vi "Voltage DAQ 07-06-2023 Current version.vi"() -> ()   [LabVIEW 2022 SP3]
uses:
  <vilib>/Utility/file.llb/Read Delimited Spreadsheet (string).vi
  <vilib>/Utility/file.llb/Write Delimited Spreadsheet (string).vi
  Labview 2018/Sub Vi's/Tektronix DPO MSO 2000 4000 Series.lvlib
panel:
  in  "Amplitude measurements":enum16{"Only test segment", "Every segment"}(ring)
  in  "Min Power (uW)":dbl=1.4
  in  "Ramping or Constant Current":enum16{"Ramping Current", "Constant Current"}(ring)
  in  "Numbers of tests":dbl
  out "Segments Run":string
  out "Power List (W)":string[](array[string])
  in  "Max Power (uW)":dbl=1200.0
  in  "Max index Seg 1 (= #Steps-1)":dbl=59.0
  out "Bandwidth":dbl[](graph)
  out "Read Buffer 2":string
  out "Read Buffer":string="+8.16433198379414E-11 ,+1.36474786384321E-14 ,+7.54655698703987E-02 ,+2.55183753967285E+01 ,+4.95928985373852E+06 ,+0.00000000000000E+00 ,+4.95929057417896E+06 ,+4.95926294501331E+06 ,+4.95931676260974E+06 \n"
  out "Local":dbl(slide) scale=0.0..100.0
  in  "Test Control":T1(ring)
  out "Ch2 Meas 2":dbl
  out "Ch1 Meas 2":dbl
  in  "Voltage Stabilize Wait (s)":dbl=1.0
  out "Ch 2 (Measurement 2)":dbl[](graph)
  out "Ch 1 (Measurement 2)":dbl[](graph)
  out "Ch2 Meas 1":dbl
  in  "Measurement 2":i32(ring)=21 items=["Period", "Frequency", "Delay", "Rise Time", "Fall Time", "Positive Duty Cycle", "Negative Duty Cycle", "Positive Pulse Width", "Negative Pulse Width", "Burst Width", "Phase", "Positive Overshoot", "Negative Overshoot", "Vpp", "Amplitude", "Voltage High", "Voltage Low", "Voltage Max", "Voltage Min", "Voltage Mean", "Voltage Mean (cycle)", "Voltage RMS", "Voltage RMS (cycle)", "Area", "Cycle Area", "Positive Edge Count", "Negative Edge Count", "Positive Pulse Count", "Negative Pulse Count", "Total Overshoot"]
  out "Ch1 Meas 1":dbl
  in  "Measurement 1":i32(ring)=13 items=["Period", "Frequency", "Delay", "Rise Time", "Fall Time", "Positive Duty Cycle", "Negative Duty Cycle", "Positive Pulse Width", "Negative Pulse Width", "Burst Width", "Phase", "Positive Overshoot", "Negative Overshoot", "Vpp", "Amplitude", "Voltage High", "Voltage Low", "Voltage Max", "Voltage Min", "Voltage Mean", "Voltage Mean (cycle)", "Voltage RMS", "Voltage RMS (cycle)", "Area", "Cycle Area", "Positive Edge Count", "Negative Edge Count", "Positive Pulse Count", "Negative Pulse Count", "Total Overshoot"]
  out "Global":u8(slide) scale=0.0..100.0
  out "Power (uW)":dbl
  out "Index (=Step#-1)":dbl=108.0
  out "Frequency":dbl[](graph)=[4959289.62588808, 4959289.85373852]
  in  "Sweep Time (s)":dbl=1.0
  in  "Step Next":bool
  in  "stop":bool
  in  "Pause":bool
  in  "Test Instructions":string="Note - DPO RESOURCE IS 11856 not 11850\nOscilloscope: Set Ch1 to 50mV (powers<80uW) or 100mV (powers between 80 and 400uW) or 200mV (powers>400uW). \nSet Ch 2 to 20 mV. \nSet trigger to 0V on  CH 1.\n"
  in  "Notes":string="Tip is 100um Stainless Steel"
  in  "Sample":string="DLC"
  in  "Sample Number":string="Box 5b Xtal 1"
  in  "Load":string="50 uN"
  in  "Tip Number":string="H10 "
  in  "Test Name":string="Ramp 3 Loc 9 test 001"
  in  "Humidity":string="2.2%"
  in  "Date":string="10/10/2022"
  in  "DPO2014 VISA Resource Name":refnum<visa-resource-name>="USB0::0x0699::0x0373::C011856::INSTR"
  in  "E5100A VISA Resource Name":refnum<visa-resource-name>="GPIB0::17::INSTR"
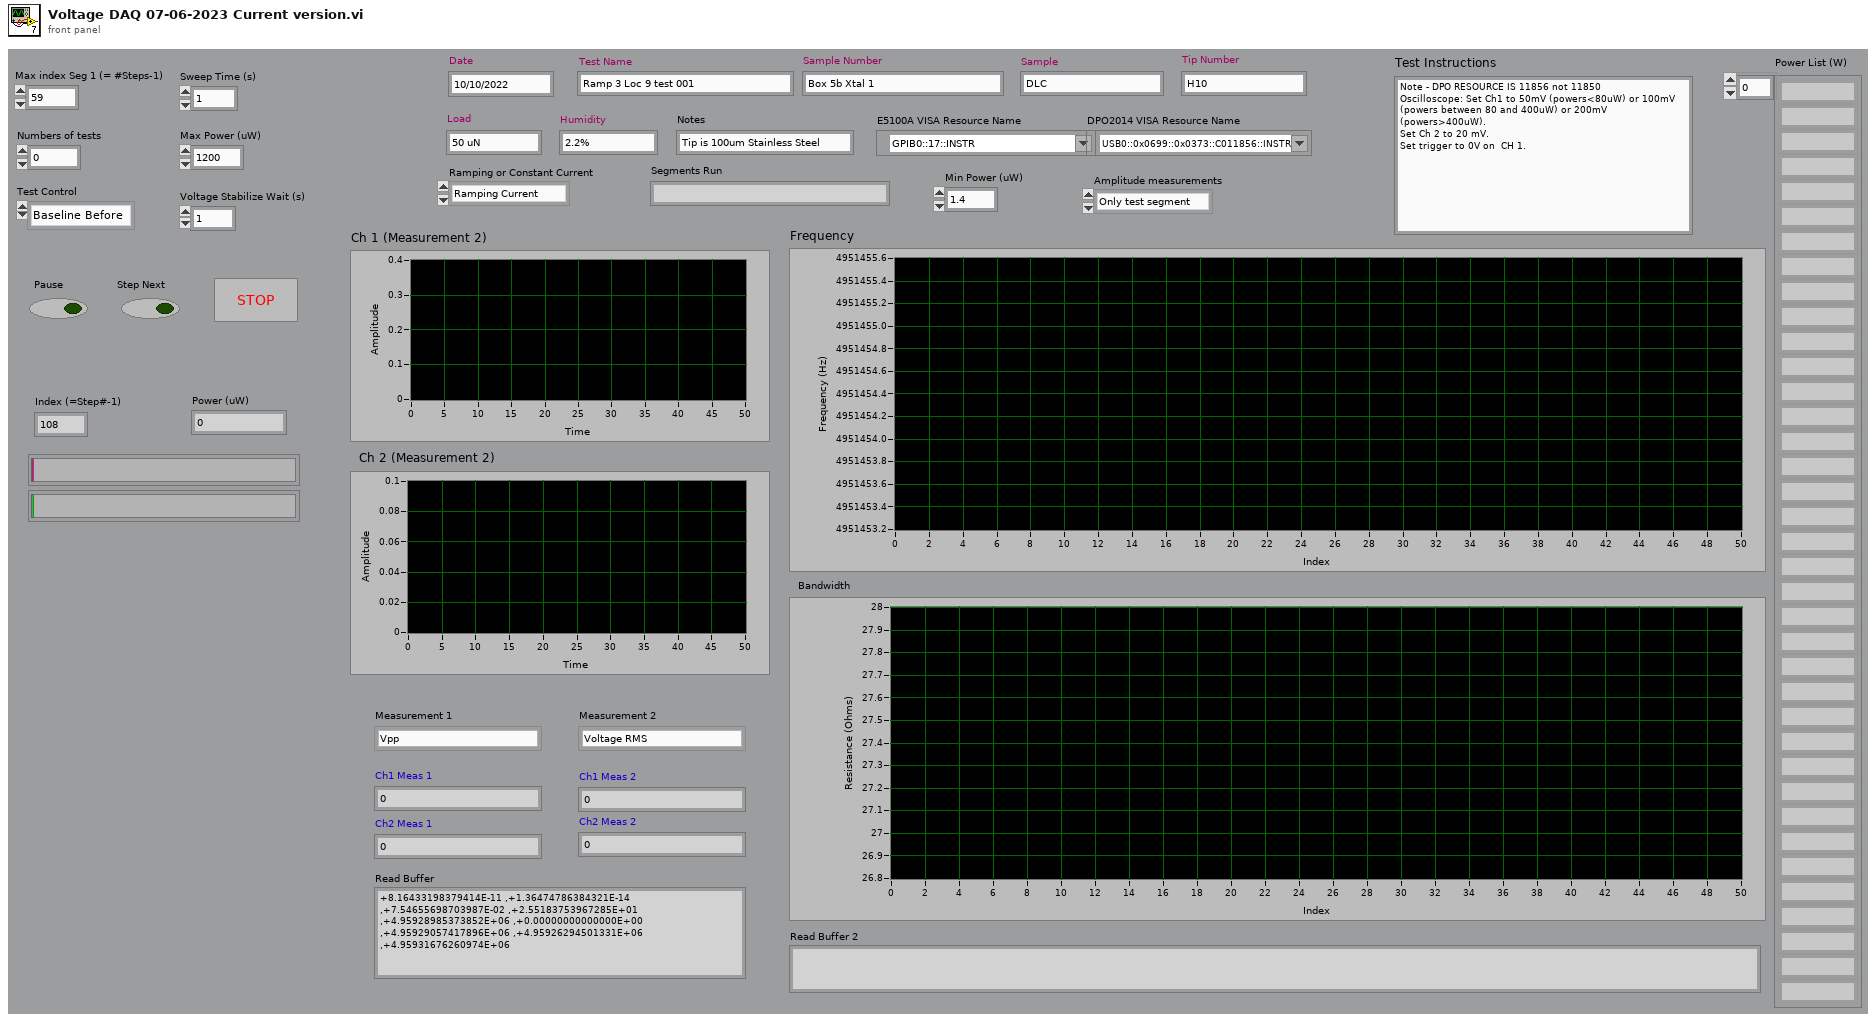
[diagram p1: front panel]
types:
  T1 = enum16{"Baseline Before", "Run-in", "Test", "Baseline After"}
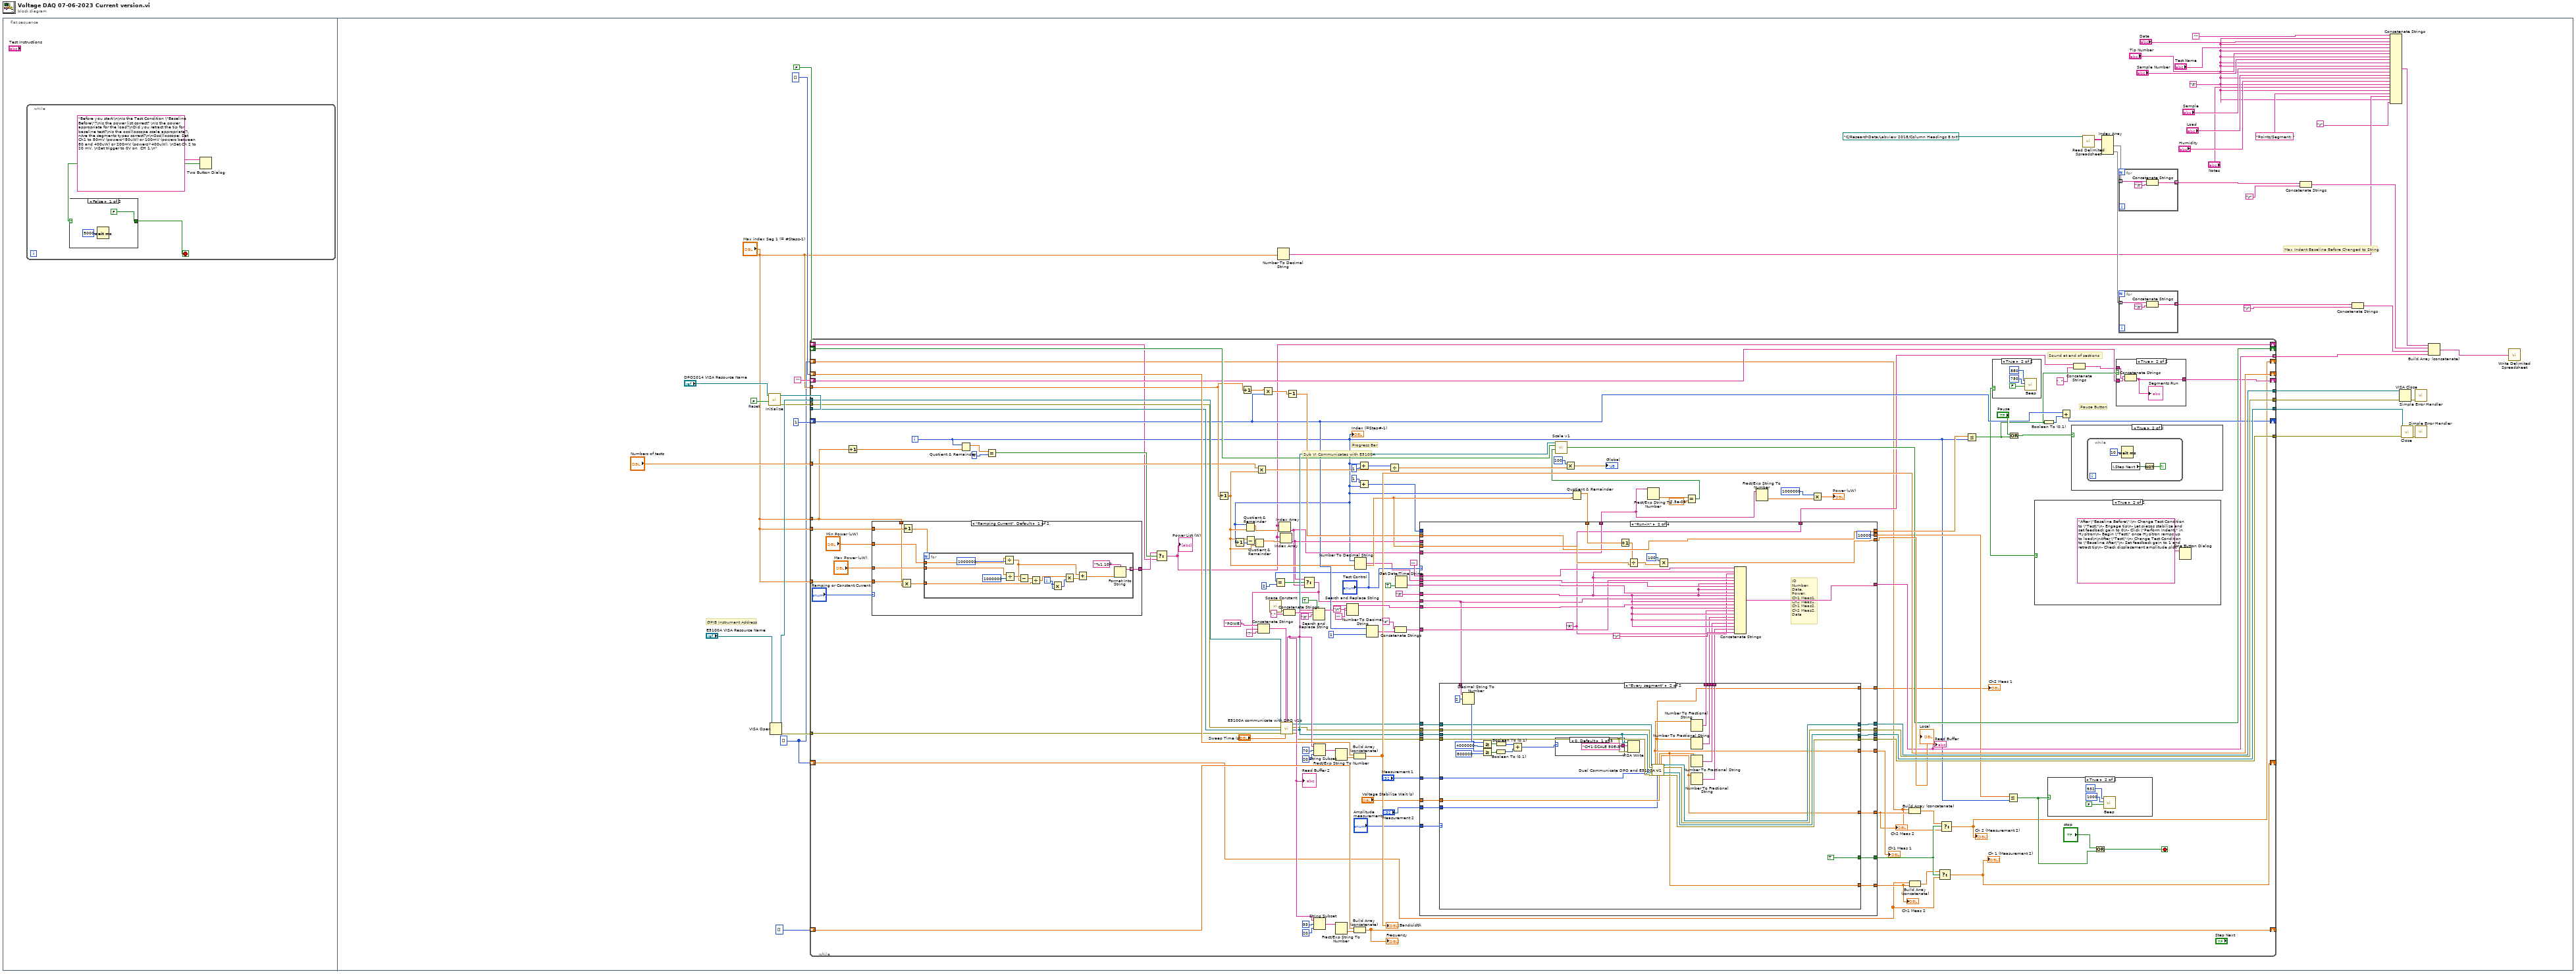
[diagram p0: block diagram]
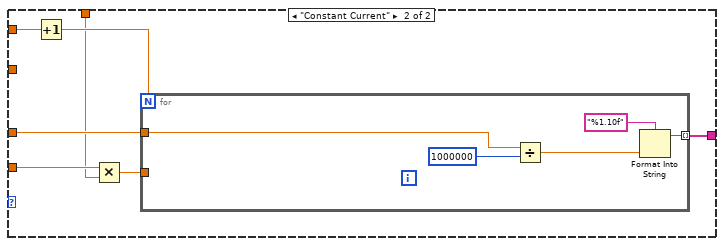
[diagram p3: hidden frame]
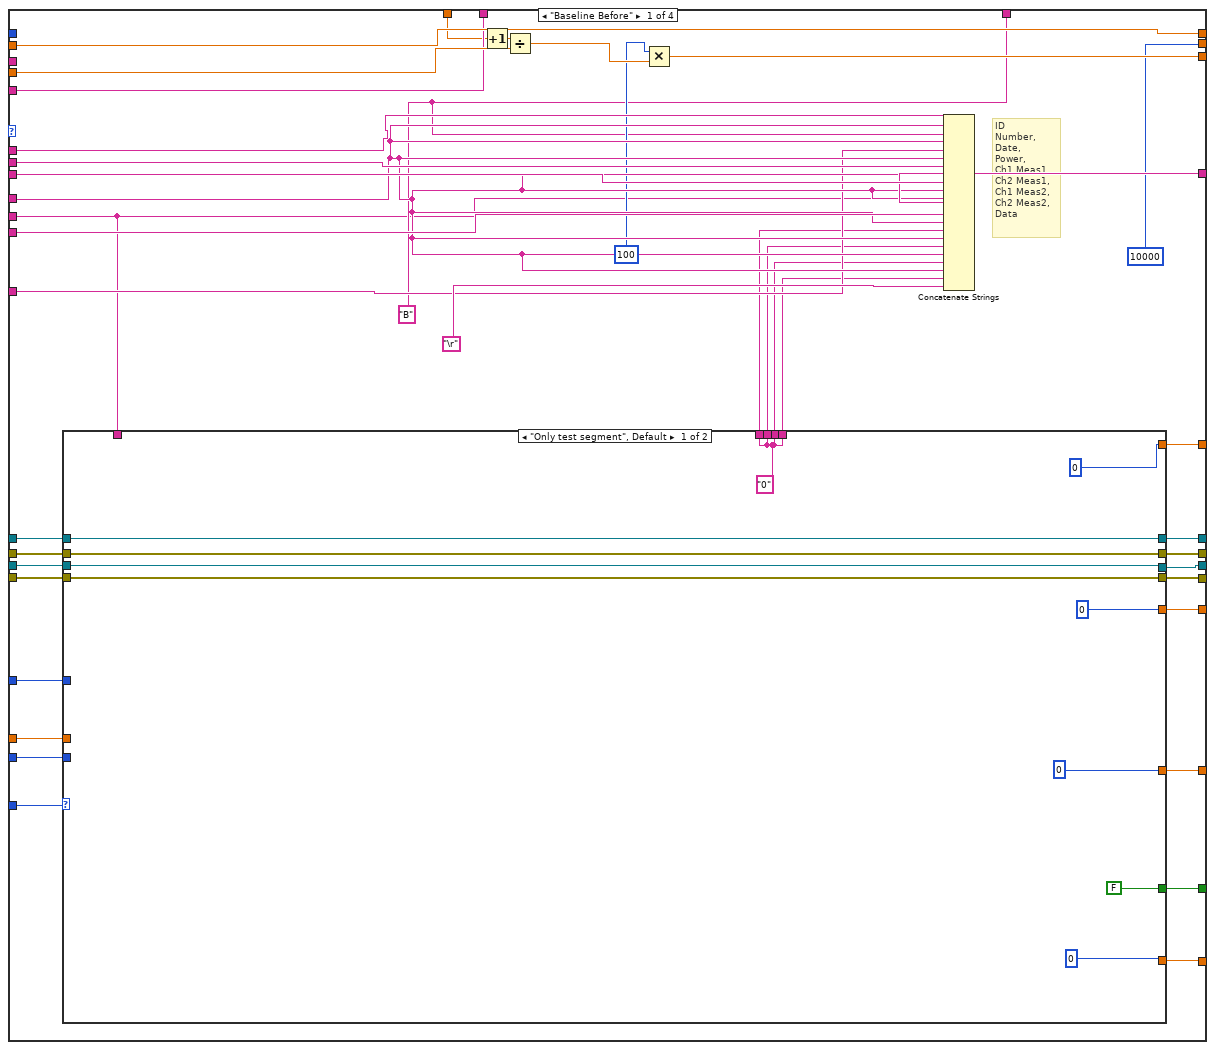
[diagram p8: hidden frame]
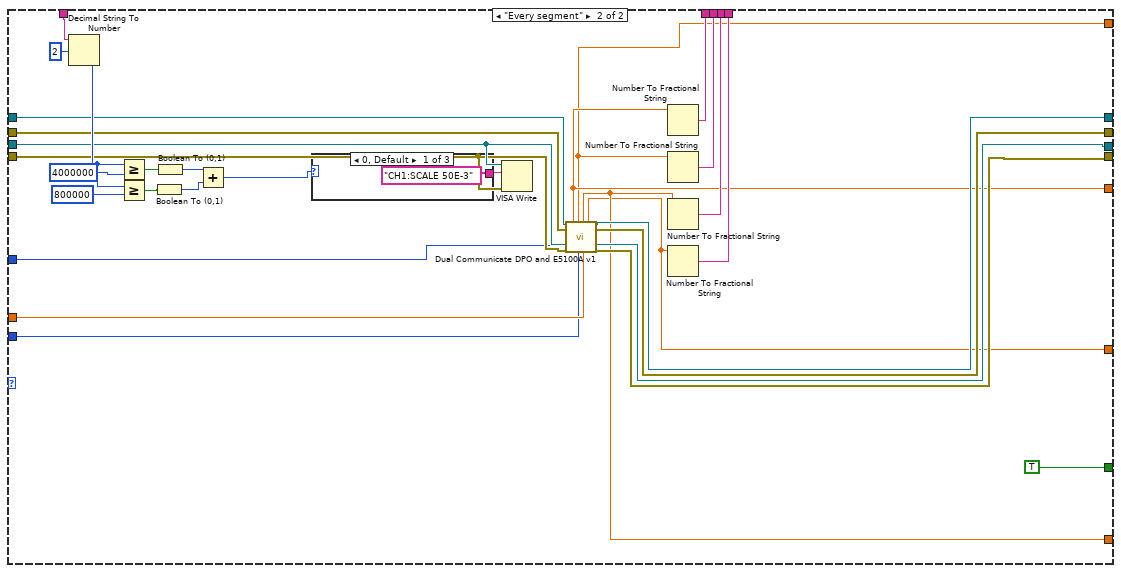
[diagram p9: hidden frame]
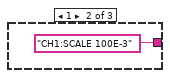
[diagram p10: hidden frame]
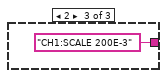
[diagram p11: hidden frame]
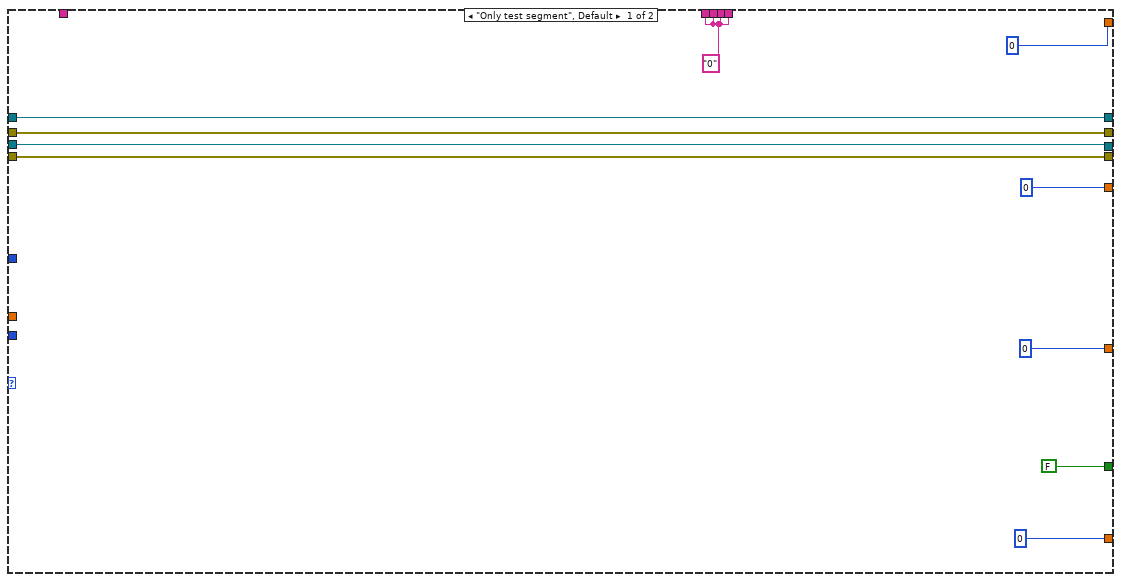
[diagram p12: hidden frame]
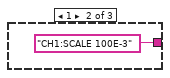
[diagram p13: hidden frame]
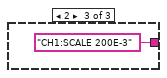
[diagram p14: hidden frame]
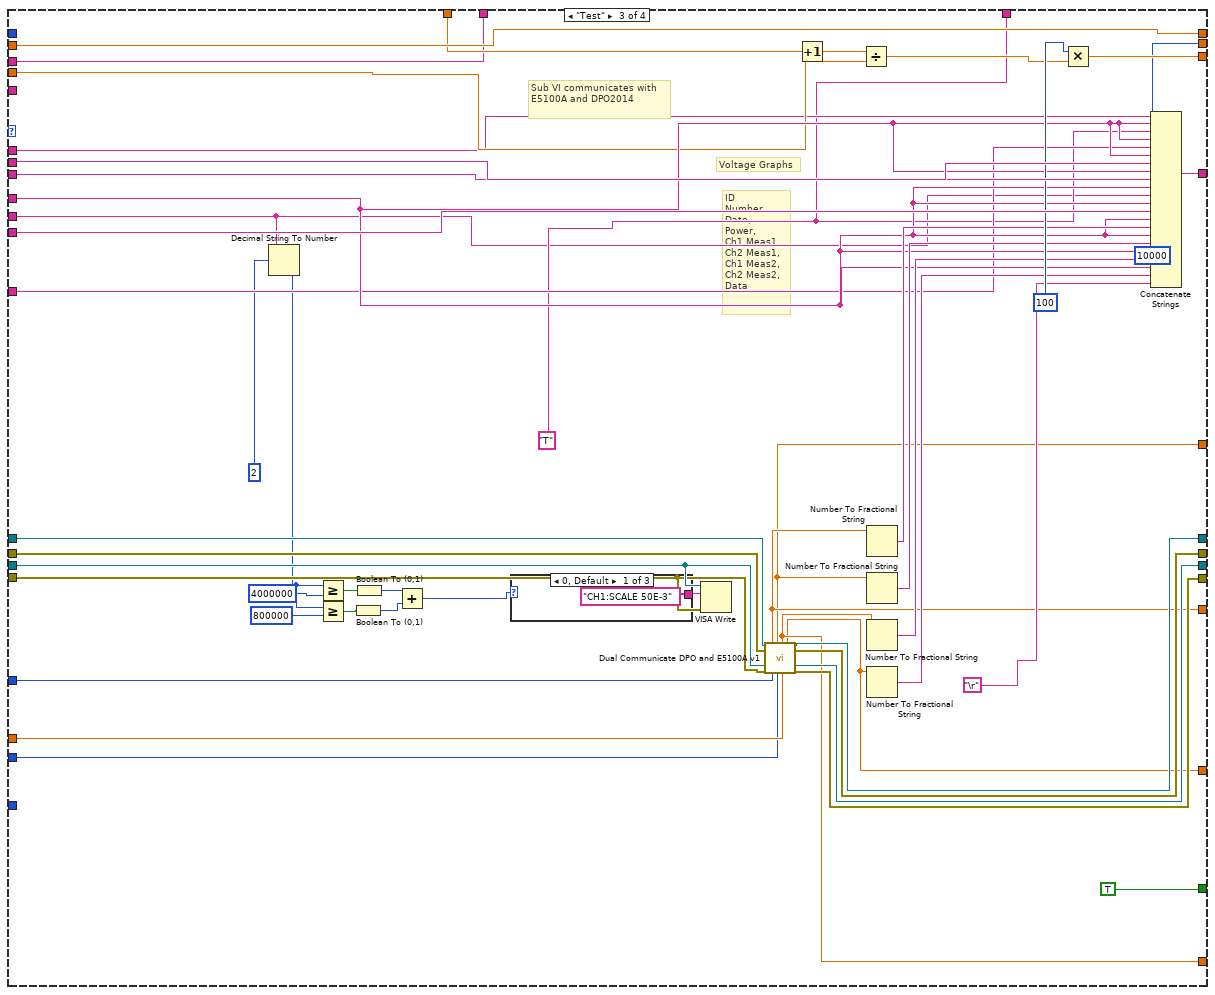
[diagram p15: hidden frame]
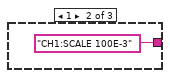
[diagram p16: hidden frame]
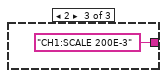
[diagram p17: hidden frame]
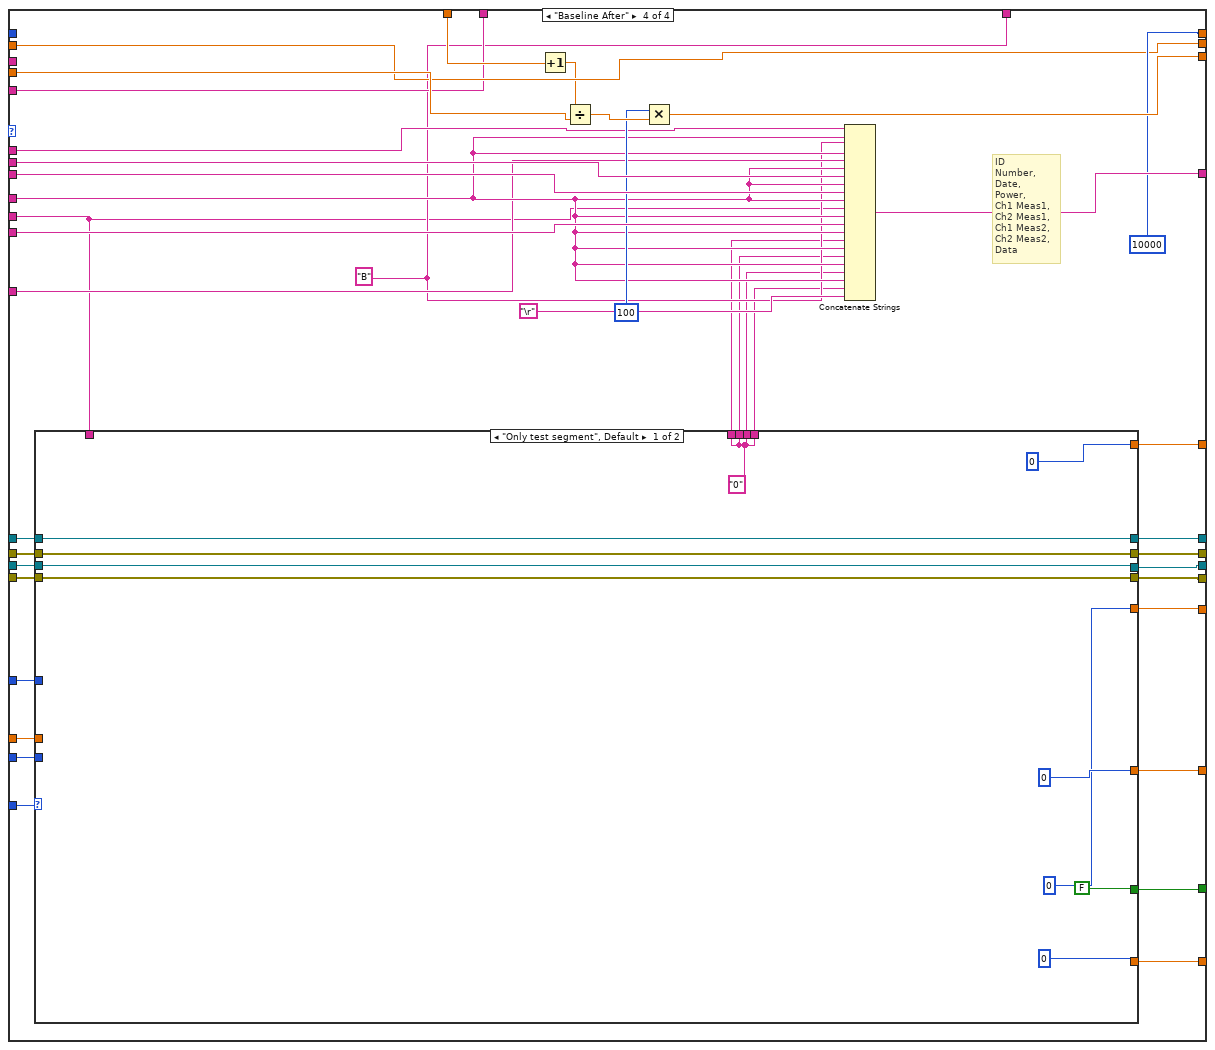
[diagram p18: hidden frame]
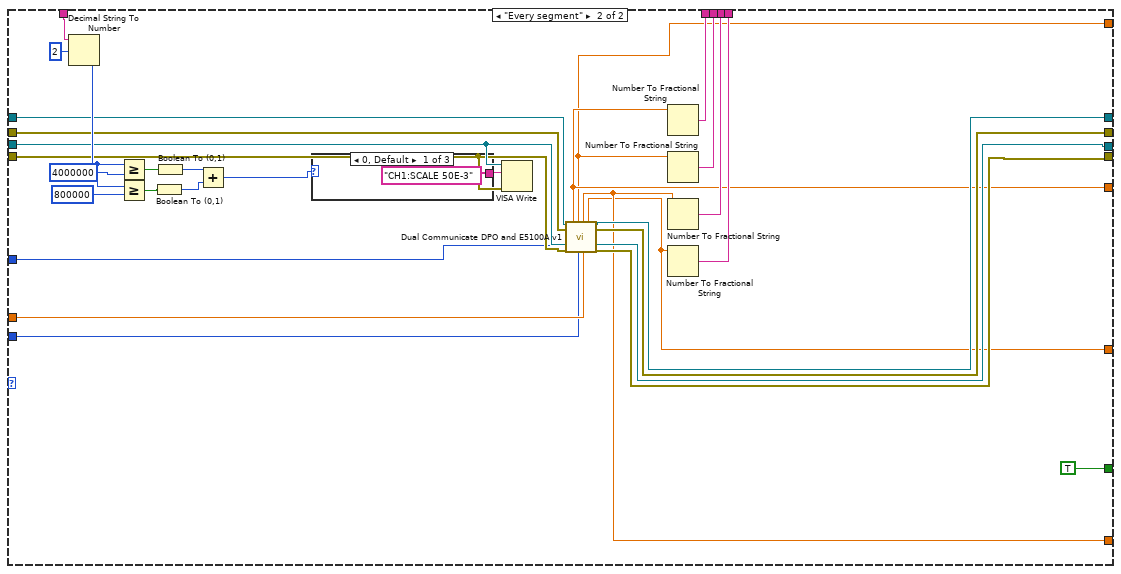
[diagram p19: hidden frame]
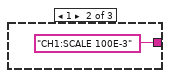
[diagram p20: hidden frame]
diagram:
  n1 = flat-sequence {
    frame #0 {
      n2 = while {
        stop <- w1 stop-if-true
        n3 = Two Button Dialog(message="Before you start:\n\nIs the Test Condition \"Baseline Before\"?\nIs the power list correct? \nIs the power appropriate for the load?\nDid you retract the tip for baseline test?\nIs the oscilloscope scale appropriate?\nAre the segments types correct?\n\nOscilloscope: Set Ch1 to 50mV (powers<80uW) or 100mV (powers between 80 and 400uW) or 200mV (powers>400uW). \nSet Ch 2 to 20 mV. \nSet trigger to 0V on  CH 1.\n") -> (T button?=w2:bool)  [unwired: 2 in]
        n4 = case shown="False" w2 {
          selector: w2 -> [_ w6]
          tunnel: [FALSE w6] -> w1
          frame False {
            n5 = Wait (ms)(milliseconds to wait=u32 5000) -> ()  [unwired: 1 out]
          }
          frame True {
          }
        }
      }
    }
    frame #1 {
      w20 = "\t" ("Tab Constant")
      w7 = i32[] []
      w17 = FALSE  # Reset
      # "Max Indent Baseline Before Changed to String"
      # "GPIB Instrument Address"
      n6 = call "Initialize.vi"("Reset (True)"=w17, "VISA resource name"="DPO2014 VISA Resource Name") -> ("error out"=w15:errorcluster, "VISA resource name out"=w8:refnum<visa-resource-name>)  [unwired: 8 in]
      n7 = VISA Open(VISA resource name="E5100A VISA Resource Name") -> (VISA resource name=w32:refnum<visa-resource-name>, error out=w33:errorcluster)  [unwired: 4 in]
      n8 = while {
        tunnel: w32 -> [w139]
        tunnel: w33 -> [w136]
        tunnel: [w168] -> w35
        tunnel: [w167] -> w36
        tunnel: w8 -> [w137]
        tunnel: w15 -> [w138]
        tunnel: [w166] -> w14
        tunnel: [w165] -> w13
        shift-right: [w60] -> _
        shift-left: w7 -> [w61]
        shift-right: [w128] -> _
        shift-left: FALSE -> [w129]
        shift-right: [w64] -> _
        shift-left: w7 -> [w63]
        shift-right: [w181] -> _
        shift-left: i32[] [] -> [w183]
        tunnel: [w140] -> w53 mode=indexing
        shift-right: [w148] -> _
        shift-left: i32[] [] -> [w149]
        tunnel: "Max index Seg 1 (= #Steps-1)" -> [w115]
        shift-right: [w145] -> _
        shift-left: 1 -> [w123]
        tunnel: "Numbers of tests" -> [w114]
        shift-right: [w96] -> _
        shift-left: "" -> [w97]
        tunnel: "Max index Seg 1 (= #Steps-1)" -> [w92]
        tunnel: "Max index Seg 1 (= #Steps-1)" -> [w91]
        tunnel: "Max index Seg 1 (= #Steps-1)" -> [w86]
        shift-right: [w81] -> _
        shift-left: _ -> [w80]
        i -> [w87]
        stop <- w124 stop-if-true
        # "Sound at end of sections"
        # "Sub VI Communicates with E5100A"
        # "Progress Bar"
        # "Pause Button"
        n9 = Increment(x=w86) -> (x+1=w79:dbl)
        n10 = case shown="\"Ramping Current\", Default" "Ramping or Constant Current" {
          tunnel: w92 -> [w193 w216]
          tunnel: w91 -> [w192 w212]
          tunnel: [w191 w217] -> w82
          tunnel: "Max Power (uW)" -> [w190 w214]
          tunnel: w86 -> [w189 w211]
          tunnel: "Min Power (uW)" -> [w188 _]
          frame "Ramping Current", Default {
            n11 = Multiply(x=w192, y=w189) -> (x*y=w195:dbl)
            n12 = Increment(x=w193) -> (x+1=w194:dbl)
            n13 = for {
              N: w194 -> [_]
              tunnel: w195 -> [w208]
              tunnel: [w203] -> w191 mode=indexing
              tunnel: w190 -> [w199]
              tunnel: w188 -> [w197]
              i -> [w210]
              n14 = Divide(x=w197, y=1000000) -> (x/y=w196:dbl)
              n15 = Divide(x=w199, y=1000000) -> (x/y=w200:dbl)
              n16 = Subtract(x=w200, y=w196) -> (x-y=w209:dbl)
              n17 = Divide(x=w209, y=w208) -> (x/y=w207:dbl)
              n18 = Multiply(x=w210, y=w210) -> (x*y=w206:i32)
              n19 = Multiply(x=w207, y=w206) -> (x*y=w205:dbl)
              n20 = Add(x=w196, y=w205) -> (x+y=w204:dbl)
              n21 = Format Into String(format string="%1.10f", w204) -> (resulting string=w203:string)  [unwired: 2 in, 1 out]
            }
          }
          frame "Constant Current" {
            n22 = Increment(x=w216) -> (x+1=w215:dbl)
            n23 = Multiply(x=w212, y=w211) -> (x*y=w213:dbl)
            n24 = for {
              N: w215 -> [_]
              tunnel: w213 -> [_]
              tunnel: [w222] -> w217 mode=indexing
              tunnel: w214 -> [w219]
              n25 = Divide(x=w219, y=1000000) -> (x/y=w220:dbl)
              n26 = Format Into String(format string="%1.10f", w220) -> (resulting string=w222:string)  [unwired: 2 in, 1 out]
            }
          }
        }
        n27 = Quotient & Remainder(x=w87, y=w79) -> (x-y*floor(x/y)=w85:dbl)  [unwired: 1 out]
        n28 = Equal?(x=w85, y=0) -> (x = y?=w83:bool)
        n29 = Select(t=w82, s=w83, f=w80) -> (s? t:f=w81:string[])
        "Power List (W)" <- w81
        n30 = Increment(x=w115) -> (x+1=w111:dbl)
        n31 = Increment(x=w87) -> (x+1=w99:i32)
        n32 = Increment(x=w115) -> (x+1=w144:dbl)
        n33 = Quotient & Remainder(x=w87, y=w111) -> (x-y*floor(x/y)=w109:dbl)  [unwired: 1 out]
        n34 = Subtract(x=w111, y=w99) -> (x-y=w112:dbl)
        n35 = Quotient & Remainder(x=w112, y=w111) -> (x-y*floor(x/y)=w110:dbl)  [unwired: 1 out]
        n36 = Multiply(x=w114, y=w111) -> (x*y=w113:dbl)
        n37 = Multiply(x=w144, y=w123) -> (x*y=w143:dbl)
        n38 = call <vilib>:"Space Constant.vi"() -> ("String"=w175:string)
        n39 = Equal?(x="Test Control", y=2) -> (x = y?=w103:bool)
        n40 = Index Array(array=w81, index=w109) -> (element=w101:string)
        n41 = Index Array(array=w81, index=w110) -> (element=w102:string)
        n42 = Concatenate Strings(w175, ",") -> (w174:string)
        n43 = Decrement(x=w143) -> (x-1=w142:dbl)
        n44 = Select(t=w102, s=w103, f=w101) -> (s? t:f=w100:string)
        n45 = Concatenate Strings("POWE ", w100, "?") -> (w134:string)
        n46 = call "E5100A communicate with DPO v1b.vi"("Sweep Time (s)"="Sweep Time (s)", "Powers"=w134, "error in (no error) 2"=w136, "DPO2014 VISA Resource"=w137, "error in (no error)"=w138, "E5100A VISA Resource Name"=w139) -> ("error out 2"=w132:errorcluster, "VISA resource name out 2"=w130:refnum<visa-resource-name>, "error out"=w74:errorcluster, "VISA resource name out"=w131:refnum<visa-resource-name>, "Read Buffer"=w133:string)  [unwired: 1 in]
        "Read Buffer 2" <- w133
        n47 = Search and Replace String(replace all?=TRUE, input string=w133, search string=w174, replace string="\t") -> (result string=w171:string)  [unwired: 4 in, 3 out]
        n48 = String Subset(string=w133, offset (0)=70, length (rest)=20) -> (substring=w151:string)
        n49 = String Subset(string=w133, offset (0)=93, length (rest)=20) -> (substring=w184:string)
        n50 = Fract/Exp String To Number(string=w151) -> (number=w150:dbl)  [unwired: 3 in, 1 out]
        n51 = Fract/Exp String To Number(string=w184) -> (number=w182:dbl)  [unwired: 3 in, 1 out]
        n52 = Search and Replace String(input string=w171, search string="\n", replace string="") -> (result string=w163:string)  [unwired: 5 in, 3 out]
        n53 = Build Array (concatenate)(w149, w150) -> (w148:dbl[])
        "Bandwidth" <- w148
        n54 = Build Array (concatenate)(w183, w182) -> (w181:dbl[])
        "Frequency" <- w181
        n55 = Number To Decimal String(number=w87) -> (decimal integer string=w76:string)  [unwired: 1 in]
        n56 = Add(x=w87, y=1) -> (x+y=w156:i32)
        n57 = Add(x=1, y=w87) -> (x+y=w75:i32)
        n58 = Number To Decimal String(number=w123, width (-)=1) -> (decimal integer string=w121:string)
        n59 = Divide(x=w156, y=w113) -> (x/y=w158:dbl)
        n60 = Concatenate Strings("s", w121) -> (w119:string)
        n61 = Get Date/Time String(want seconds? (F)=TRUE) -> (time string=w77:string)  [unwired: 2 in, 1 out]
        n62 = Multiply(x=100, y=w158) -> (x*y=→"Global":dbl)
        n63 = Quotient & Remainder(x=w87, y=w111) -> (x-y*floor(x/y)=w116:dbl)  [unwired: 1 out]
        n64 = case shown="\"Run-in\"" "Test Control" {
          tunnel: [w248 w337 w436 w470] -> w168
          tunnel: [w249 w335 w435 w469] -> w167
          tunnel: [w250 w331 w434 w468] -> w166
          tunnel: [w251 w332 w433 w467] -> w165
          tunnel: "" -> [w263 w347 w432 w483]
          tunnel: w76 -> [w273 w351 w450 w493]
          tunnel: "\t" -> [w265 w349 w438 w485]
          tunnel: w77 -> [w272 w348 w449 w492]
          tunnel: w163 -> [w271 w350 w448 w491]
          tunnel: [w270 w353 w447 w490] -> w140
          tunnel: w111 -> [w267 w352 w437 w484]
          tunnel: [w268 w354 w444 w487] -> w161
          tunnel: w75 -> [_ _ _ _]
          tunnel: w142 -> [w264 w344 w429 w480]
          tunnel: [w264 w344 w429 10000] -> w141
          tunnel: w131 -> [w255 w338 w423 w472]
          tunnel: w74 -> [w254 w336 w422 w473]
          tunnel: w130 -> [w252 w334 w421 w474]
          tunnel: w132 -> [w253 w333 w420 w475]
          tunnel: [10000 10000 10000 w480] -> w127
          tunnel: w119 -> [w261 w345 w430 w481]
          tunnel: w101 -> [w259 w341 _ w477]
          tunnel: w116 -> [w257 w342 w427 w478]
          tunnel: [w259 w341 w426 w477] -> w107
          tunnel: w102 -> [_ _ w426 _]
          tunnel: w100 -> [w242 w330 w419 w471]
          tunnel: [w258 w340 w425 w476] -> w93
          tunnel: "Amplitude measurements" -> [w243 w339 _ w462]
          tunnel: "Voltage Stabilize Wait (s)" -> [w241 w325 w409 w460]
          tunnel: "Measurement 1" -> [w240 w323 w408 w461]
          tunnel: "Measurement 2" -> [w239 w324 w407 w459]
          tunnel: [w238 w322 w406 w458] -> w70
          tunnel: [w237 w321 w403 w457] -> w67
          tunnel: [w236 w320 w405 w456] -> w69
          tunnel: [w235 w319 w404 w455] -> w68
          tunnel: [w234 w318 TRUE w454] -> w66
          frame "Baseline Before" {
            w258 = "B"
            # "ID\nNumber,\nDate,\nPower,\nCh1 Meas1,\nCh2 Meas1,\nCh1 Meas2,\nCh2 Meas2,\nData"
            n65 = case shown="\"Only test segment\", Default" w243 {
              tunnel: [w283 w301] -> w248
              tunnel: w255 -> [w283 w305]
              tunnel: w254 -> [w282 w304]
              tunnel: [w282 w300] -> w249
              tunnel: [w281 w299] -> w250
              tunnel: w252 -> [w281 w303]
              tunnel: [w280 w298] -> w251
              tunnel: w253 -> [w280 w302]
              tunnel: w242 -> [_ w296]
              tunnel: [w279 w295] -> w247
              tunnel: [w279 w294] -> w246
              tunnel: [w279 w293] -> w245
              tunnel: [w279 w292] -> w244
              tunnel: [0 w285] -> w235
              tunnel: [0 w291] -> w236
              tunnel: [0 w290] -> w238
              tunnel: [0 w289] -> w237
              tunnel: w241 -> [_ w288]
              tunnel: w240 -> [_ w287]
              tunnel: w239 -> [_ w286]
              tunnel: [FALSE TRUE] -> w234
              frame "Only test segment", Default {
                w279 = "0"
              }
              frame "Every segment" {
                n66 = Decimal String To Number(string=w296, offset=2) -> (number=w311:i32)  [unwired: 1 in, 1 out]
                n67 = Greater Or Equal?(x=w311, y=4000000) -> (x >= y?=w310:bool)
                n68 = Greater Or Equal?(x=w311, y=800000) -> (x >= y?=w309:bool)
                n69 = Boolean To (0,1)(Boolean=w309) -> (0, 1=w307:i16)
                n70 = Boolean To (0,1)(Boolean=w310) -> (0, 1=w308:i16)
                n71 = Add(x=w308, y=w307) -> (x+y=w306:i16)
                n72 = case shown="0, Default" w306 {
                  tunnel: ["CH1:SCALE 50E-3" "CH1:SCALE 100E-3" "CH1:SCALE 200E-3"] -> w314
                  frame 0, Default {
                  }
                  frame 1 {
                  }
                  frame 2 {
                  }
                }
                n73 = VISA Write(VISA resource name=w303, write buffer=w314, error in (no error)=w302) -> ()  [unwired: 3 out]
                n74 = call "Dual Communicate DPO and E5100A v1.vi"("E5100A VISA Resource Name"=w305, "error in (no error)"=w304, "DPO2014 VISA Resource Name"=w303, "error in (no error) 2"=w302, "Measurement Function 1"=w287, "Measurement Function 2"=w286, "Voltage Stabilize Wait (s)"=w288) -> ("Measurement Value 1"=w291:dbl, "Measurement Value 2"=w285:dbl, "Measurement Value 3"=w290:dbl, "Measurement Value 4"=w289:dbl, "VISA resource name out"=w301:refnum<visa-resource-name>, "error out"=w300:errorcluster, "VISA resource name out 2"=w299:refnum<visa-resource-name>, "error out 2"=w298:errorcluster)  [unwired: 5 in]
                n75 = Number To Fractional String(number=w291) -> (F-format string=w292:string)  [unwired: 3 in]
                n76 = Number To Fractional String(number=w285) -> (F-format string=w293:string)  [unwired: 3 in]
                n77 = Number To Fractional String(number=w290) -> (F-format string=w294:string)  [unwired: 3 in]
                n78 = Number To Fractional String(number=w289) -> (F-format string=w295:string)  [unwired: 3 in]
              }
            }
            n79 = Increment(x=w257) -> (x+1=w256:dbl)
            n80 = Divide(x=w256, y=w267) -> (x/y=w269:dbl)
            n81 = Multiply(x=100, y=w269) -> (x*y=w268:dbl)
            n82 = Concatenate Strings(w263, w265, w258, w265, w261, w265, w273, w265, w272, w265, w242, w265, w271, w265, w244, w265, w245, w265, w246, w265, w247, "\r") -> (w270:string)
          }
          frame "Run-in" {
            w340 = "R"
            # "ID\nNumber,\nDate,\nPower,\nCh1 Meas1,\nCh2 Meas1,\nCh1 Meas2,\nCh2 Meas2,\nData"
            n83 = case shown="\"Every segment\"" w339 {
              tunnel: [w367 w385] -> w337
              tunnel: w338 -> [w367 w389]
              tunnel: w336 -> [w366 w388]
              tunnel: [w366 w384] -> w335
              tunnel: [w365 w383] -> w331
              tunnel: w334 -> [w365 w387]
              tunnel: [w364 w382] -> w332
              tunnel: w333 -> [w364 w386]
              tunnel: w330 -> [_ w380]
              tunnel: [w363 w379] -> w329
              tunnel: [w363 w378] -> w328
              tunnel: [w363 w377] -> w327
              tunnel: [w363 w376] -> w326
              tunnel: w325 -> [_ w375]
              tunnel: w324 -> [_ w374]
              tunnel: w323 -> [_ w373]
              tunnel: [0 w372] -> w322
              tunnel: [0 w369] -> w319
              tunnel: [0 w371] -> w320
              tunnel: [0 w370] -> w321
              tunnel: [FALSE TRUE] -> w318
              frame "Only test segment", Default {
                w363 = "0"
              }
              frame "Every segment" {
                n84 = Decimal String To Number(string=w380, offset=2) -> (number=w395:i32)  [unwired: 1 in, 1 out]
                n85 = Greater Or Equal?(x=w395, y=4000000) -> (x >= y?=w394:bool)
                n86 = Greater Or Equal?(x=w395, y=800000) -> (x >= y?=w393:bool)
                n87 = Boolean To (0,1)(Boolean=w393) -> (0, 1=w391:i16)
                n88 = Boolean To (0,1)(Boolean=w394) -> (0, 1=w392:i16)
                n89 = Add(x=w392, y=w391) -> (x+y=w390:i16)
                n90 = case shown="0, Default" w390 {
                  tunnel: ["CH1:SCALE 50E-3" "CH1:SCALE 100E-3" "CH1:SCALE 200E-3"] -> w398
                  frame 0, Default {
                  }
                  frame 1 {
                  }
                  frame 2 {
                  }
                }
                n91 = VISA Write(VISA resource name=w387, write buffer=w398, error in (no error)=w386) -> ()  [unwired: 3 out]
                n92 = call "Dual Communicate DPO and E5100A v1.vi"("E5100A VISA Resource Name"=w389, "error in (no error)"=w388, "DPO2014 VISA Resource Name"=w387, "error in (no error) 2"=w386, "Measurement Function 1"=w373, "Measurement Function 2"=w374, "Voltage Stabilize Wait (s)"=w375) -> ("Measurement Value 1"=w371:dbl, "Measurement Value 2"=w369:dbl, "Measurement Value 3"=w372:dbl, "Measurement Value 4"=w370:dbl, "VISA resource name out"=w385:refnum<visa-resource-name>, "error out"=w384:errorcluster, "VISA resource name out 2"=w383:refnum<visa-resource-name>, "error out 2"=w382:errorcluster)  [unwired: 5 in]
                n93 = Number To Fractional String(number=w371) -> (F-format string=w376:string)  [unwired: 3 in]
                n94 = Number To Fractional String(number=w369) -> (F-format string=w377:string)  [unwired: 3 in]
                n95 = Number To Fractional String(number=w372) -> (F-format string=w378:string)  [unwired: 3 in]
                n96 = Number To Fractional String(number=w370) -> (F-format string=w379:string)  [unwired: 3 in]
              }
            }
            n97 = Increment(x=w342) -> (x+1=w343:dbl)
            n98 = Divide(x=w343, y=w352) -> (x/y=w357:dbl)
            n99 = Multiply(x=100, y=w357) -> (x*y=w354:dbl)
            n100 = Concatenate Strings(w347, w349, w340, w349, w345, w349, w351, w349, w348, w349, w330, w349, w350, w349, w326, w349, w327, w349, w328, w349, w329, "\r") -> (w353:string)
          }
          frame "Test" {
            w425 = "T"
            # "Sub VI communicates with E5100A and DPO2014"
            # "Voltage Graphs"
            # "ID\nNumber,\nDate,\nPower,\nCh1 Meas1,\nCh2 Meas1,\nCh1 Meas2,\nCh2 Meas2,\nData"
            n101 = Decimal String To Number(string=w419, offset=2) -> (number=w416:i32)  [unwired: 1 in, 1 out]
            n102 = Greater Or Equal?(x=w416, y=4000000) -> (x >= y?=w415:bool)
            n103 = Greater Or Equal?(x=w416, y=800000) -> (x >= y?=w414:bool)
            n104 = Boolean To (0,1)(Boolean=w414) -> (0, 1=w412:i16)
            n105 = Boolean To (0,1)(Boolean=w415) -> (0, 1=w413:i16)
            n106 = Add(x=w413, y=w412) -> (x+y=w411:i16)
            n107 = case shown="0, Default" w411 {
              tunnel: ["CH1:SCALE 50E-3" "CH1:SCALE 100E-3" "CH1:SCALE 200E-3"] -> w424
              frame 0, Default {
              }
              frame 1 {
              }
              frame 2 {
              }
            }
            n108 = VISA Write(VISA resource name=w421, write buffer=w424, error in (no error)=w420) -> ()  [unwired: 3 out]
            n109 = call "Dual Communicate DPO and E5100A v1.vi"("E5100A VISA Resource Name"=w423, "error in (no error)"=w422, "DPO2014 VISA Resource Name"=w421, "error in (no error) 2"=w420, "Measurement Function 1"=w408, "Measurement Function 2"=w407, "Voltage Stabilize Wait (s)"=w409) -> ("Measurement Value 1"=w405:dbl, "Measurement Value 2"=w404:dbl, "Measurement Value 3"=w406:dbl, "Measurement Value 4"=w403:dbl, "VISA resource name out"=w436:refnum<visa-resource-name>, "error out"=w435:errorcluster, "VISA resource name out 2"=w434:refnum<visa-resource-name>, "error out 2"=w433:errorcluster)  [unwired: 5 in]
            n110 = Increment(x=w427) -> (x+1=w428:dbl)
            n111 = Divide(x=w428, y=w437) -> (x/y=w445:dbl)
            n112 = Number To Fractional String(number=w405) -> (F-format string=w440:string)  [unwired: 3 in]
            n113 = Number To Fractional String(number=w404) -> (F-format string=w441:string)  [unwired: 3 in]
            n114 = Number To Fractional String(number=w406) -> (F-format string=w442:string)  [unwired: 3 in]
            n115 = Number To Fractional String(number=w403) -> (F-format string=w443:string)  [unwired: 3 in]
            n116 = Multiply(x=100, y=w445) -> (x*y=w444:dbl)
            n117 = Concatenate Strings(w432, w438, w425, w438, w430, w438, w450, w438, w449, w438, w419, w438, w448, w438, w440, w438, w441, w438, w442, w438, w443, "\r") -> (w447:string)
          }
          frame "Baseline After" {
            w476 = "B"
            # "ID\nNumber,\nDate,\nPower,\nCh1 Meas1,\nCh2 Meas1,\nCh1 Meas2,\nCh2 Meas2,\nData"
            n118 = case shown="\"Only test segment\", Default" w462 {
              tunnel: [w503 w521] -> w470
              tunnel: w472 -> [w503 w525]
              tunnel: w473 -> [w502 w524]
              tunnel: [w502 w520] -> w469
              tunnel: [w501 w519] -> w468
              tunnel: w474 -> [w501 w523]
              tunnel: [w500 w518] -> w467
              tunnel: w475 -> [w500 w522]
              tunnel: w471 -> [_ w516]
              tunnel: [w499 w515] -> w466
              tunnel: [w499 w514] -> w465
              tunnel: [w499 w513] -> w464
              tunnel: [w499 w512] -> w463
              tunnel: [0 w507] -> w458
              tunnel: [0 w511] -> w456
              tunnel: [0 w505] -> w455
              tunnel: w461 -> [_ w510]
              tunnel: w460 -> [_ w509]
              tunnel: w459 -> [_ w508]
              tunnel: [0 w506] -> w457
              tunnel: [FALSE TRUE] -> w454
              frame "Only test segment", Default {
                w499 = "0"
              }
              frame "Every segment" {
                n119 = Decimal String To Number(string=w516, offset=2) -> (number=w531:i32)  [unwired: 1 in, 1 out]
                n120 = Greater Or Equal?(x=w531, y=4000000) -> (x >= y?=w530:bool)
                n121 = Greater Or Equal?(x=w531, y=800000) -> (x >= y?=w529:bool)
                n122 = Boolean To (0,1)(Boolean=w529) -> (0, 1=w527:i16)
                n123 = Boolean To (0,1)(Boolean=w530) -> (0, 1=w528:i16)
                n124 = Add(x=w528, y=w527) -> (x+y=w526:i16)
                n125 = case shown="0, Default" w526 {
                  tunnel: ["CH1:SCALE 50E-3" "CH1:SCALE 100E-3" "CH1:SCALE 200E-3"] -> w534
                  frame 0, Default {
                  }
                  frame 1 {
                  }
                  frame 2 {
                  }
                }
                n126 = VISA Write(VISA resource name=w523, write buffer=w534, error in (no error)=w522) -> ()  [unwired: 3 out]
                n127 = call "Dual Communicate DPO and E5100A v1.vi"("E5100A VISA Resource Name"=w525, "error in (no error)"=w524, "DPO2014 VISA Resource Name"=w523, "error in (no error) 2"=w522, "Measurement Function 1"=w510, "Measurement Function 2"=w508, "Voltage Stabilize Wait (s)"=w509) -> ("Measurement Value 1"=w511:dbl, "Measurement Value 2"=w505:dbl, "Measurement Value 3"=w507:dbl, "Measurement Value 4"=w506:dbl, "VISA resource name out"=w521:refnum<visa-resource-name>, "error out"=w520:errorcluster, "VISA resource name out 2"=w519:refnum<visa-resource-name>, "error out 2"=w518:errorcluster)  [unwired: 5 in]
                n128 = Number To Fractional String(number=w511) -> (F-format string=w512:string)  [unwired: 3 in]
                n129 = Number To Fractional String(number=w505) -> (F-format string=w513:string)  [unwired: 3 in]
                n130 = Number To Fractional String(number=w507) -> (F-format string=w514:string)  [unwired: 3 in]
                n131 = Number To Fractional String(number=w506) -> (F-format string=w515:string)  [unwired: 3 in]
              }
            }
            n132 = Increment(x=w478) -> (x+1=w479:dbl)
            n133 = Divide(x=w479, y=w484) -> (x/y=w489:dbl)
            n134 = Multiply(x=100, y=w489) -> (x*y=w487:dbl)
            n135 = Concatenate Strings(w483, w485, w476, w485, w481, w485, w493, w485, w492, w485, w471, w485, w491, w485, w463, w485, w464, w485, w465, w485, w466, "\r") -> (w490:string)
          }
        }
        "Local" <- w161
        "Read Buffer" <- w140
        "Ch1 Meas 2" <- w70
        "Ch2 Meas 2" <- w67
        "Ch1 Meas 1" <- w69
        "Ch2 Meas 1" <- w68
        n136 = Fract/Exp String To Number(string=w107) -> (number=w118:dbl)  [unwired: 3 in, 1 out]
        n137 = Equal?(x=w118, y=7.5e-05) -> (x = y?=w108:bool)
        n138 = call "Scale v1.vi"("Right Power?"=w108, "Global True False"=w129, "VISA resource name"=w130) -> ("Boolean"=w128:bool)  [unwired: 3 in]
        n139 = Fract/Exp String To Number(string=w107) -> (number=w178:dbl)  [unwired: 3 in, 1 out]
        n140 = Multiply(x=1000000, y=w178) -> (x*y=→"Power (uW)":dbl)
        n141 = Build Array (concatenate)(w63, w67) -> (w65:dbl[])
        n142 = Build Array (concatenate)(w61, w70) -> (w62:dbl[])
        n143 = Select(t=w62, s=w66, f=w61) -> (s? t:f=w60:dbl[])
        "Ch 1 (Measurement 2)" <- w60
        n144 = Select(t=w65, s=w66, f=w63) -> (s? t:f=w64:dbl[])
        "Ch 2 (Measurement 2)" <- w64
        n145 = Less Or Equal?(x=w141, y=w87) -> (x <= y?=w98:bool)
        n146 = case shown="True" w98 {
          frame False {
          }
          frame True {
            n147 = call <vilib>:"Beep.vi"("use system alert? (T)"=FALSE, "duration (msec)"=750, "frequency (Hz)"=880) -> ()  [unwired: 9 in]
          }
        }
        n148 = Less Or Equal?(x=w127, y=w87) -> (x <= y?=w126:bool)
        n149 = Or(x="Pause", y=w98) -> (x .or. y?=w159:bool)
        n150 = case shown="True" w98 {
          frame False {
          }
          frame True {
            n151 = One Button Dialog(message="After \"Baseline Before\":\n- Change Test Condition to \"Test\"\n- Engage tip\n- Let piezos stabilize and set feedback gain to 0\n- Click \"Perform Indent\" in Hysitron\n- Begin \"Test\" once Hysitron ramps up to load\n\nAfter \"Test\":\n- Change Test Condition to \"Baseline After\"\n- Set feedback gain to 1 and retract tip\n- Check displacement amplitude plot") -> ()  [unwired: 1 in, 1 out]
          }
        }
        n152 = Boolean To (0,1)(Boolean=w98) -> (0, 1=w146:i16)
        n153 = case shown="True" w126 {
          frame False {
          }
          frame True {
            n154 = call <vilib>:"Beep.vi"("use system alert? (T)"=FALSE, "duration (msec)"=1000, "frequency (Hz)"=932) -> ()  [unwired: 9 in]
          }
        }
        n155 = Add(x=w123, y=w146) -> (x+y=w145:i32)
        n156 = case shown="True" w159 {
          frame False {
          }
          frame True {
            n157 = while {
              stop <- w538 continue-if-true
              n158 = local read "Step Next"() -> (w539:bool)
              n159 = Wait (ms)(milliseconds to wait=u32 10) -> ()  [unwired: 1 out]
              n160 = Not(x=w539) -> (.not. x?=w538:bool)
            }
          }
        }
        n161 = Concatenate Strings(w93, ", ") -> (w95:string)
        n162 = Or(x="stop", y=w126) -> (x .or. y?=w124:bool)
        n163 = case shown="True" w98 {
          tunnel: w97 -> [w223 w225]
          tunnel: [w223 w226] -> w96
          tunnel: w95 -> [_ w224]
          frame False {
          }
          frame True {
            n164 = Concatenate Strings(w225, w224) -> (w226:string)
            "Segments Run" <- w226
          }
        }
        "Index (=Step#-1)" <- w87
      }
      n165 = Number To Decimal String(number="Max index Seg 1 (= #Steps-1)") -> (decimal integer string=w21:string)  [unwired: 1 in]
      n166 = call-poly <vilib>:"Read Delimited Spreadsheet.vi"("file path (dialog if empty)"=path "C:/ResearchData/Labview 2018/Column Headings 8.txt") -> ("all rows"=w44:string[][])  [unwired: 9 in, 5 out]
      n167 = Index Array(array=w44) -> (element #1=w51:string[], element #2=w49:string[])  [unwired: 4 in]
      n168 = for {
        tunnel: w51 -> [w56] mode=indexing
        tunnel: [w54] -> w52 mode=indexing
        n169 = Concatenate Strings(w56, "\t") -> (w54:string)
      }
      n170 = for {
        tunnel: w49 -> [w59] mode=indexing
        tunnel: [w57] -> w50 mode=indexing
        n171 = Concatenate Strings(w59, "\t") -> (w57:string)
      }
      n172 = Concatenate Strings(w52, "\r") -> (w47:string)
      n173 = Concatenate Strings(w50, "\r") -> (w48:string)
      n174 = Concatenate Strings "Concatenate Strings"("", w20, "Date", w20, "Test Name", w20, "Tip Number", w20, "Sample Number", w20, w20, "Sample", w20, "Load", w20, "Humidity", w20, "Notes", w20, "Points/Segment: ", w21, w20, "\r") -> (w46:string)
      n175 = VISA Close(VISA resource name=w35, error in (no error)=w36) -> (error out=w34:errorcluster)
      n176 = call "Close.vi"("error in (no error)"=w13, "VISA resource name"=w14) -> ("error out"=w12:errorcluster)  [unwired: 9 in]
      n177 = call <vilib>:"Simple Error Handler.vi"("error in (no error)"=w34) -> ()  [unwired: 4 in, 5 out]
      n178 = call <vilib>:"Simple Error Handler.vi"("error in (no error)"=w12) -> ()  [unwired: 4 in, 5 out]
      n179 = Build Array (concatenate) "Build Array"(w46, w47, w48, w53) -> (w45:string[])
      n180 = call-poly <vilib>:"Write Delimited Spreadsheet.vi"("1D data"=w45) -> ()  [unwired: 13 in, 2 out]
    }
  }
